vi "DestroyClone.vi"(8 "error in (no error)":errorcluster, 9 "Exit via Stop Module Req?":bool, 10 "Wait for Module to stop?":bool, 11 "ModuleAdmin":refnum<class "ModuleAdmin.lvclass">) -> (0 "error out":errorcluster, 1 "External Launch":bool, 3 "Mod Admin out":refnum<class "ModuleAdmin.lvclass">)   [LabVIEW 2014, in "PmuImpairModule.lvlib"]
uses:
  PmuImpairModule.lvlib
  <userlib>/NIST/ModuleAdminLib/ModuleAdmin/ModuleAdmin.lvclass
  <userlib>/NIST/ModuleAdminLib/ModuleAdmin/ModuleAdmin.lvclass/ModuleAdmin.ctl
  <userlib>/NIST/ModuleAdminLib/ModuleAdmin/Accessors/Read CloneRegRef.vi
  <userlib>/NIST/ModuleAdminLib/CloneRegistration/CloneRegistration.lvclass
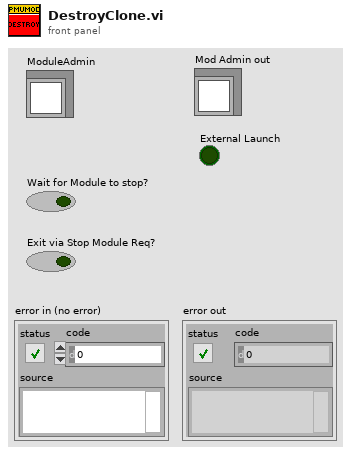
[diagram p1: front panel]
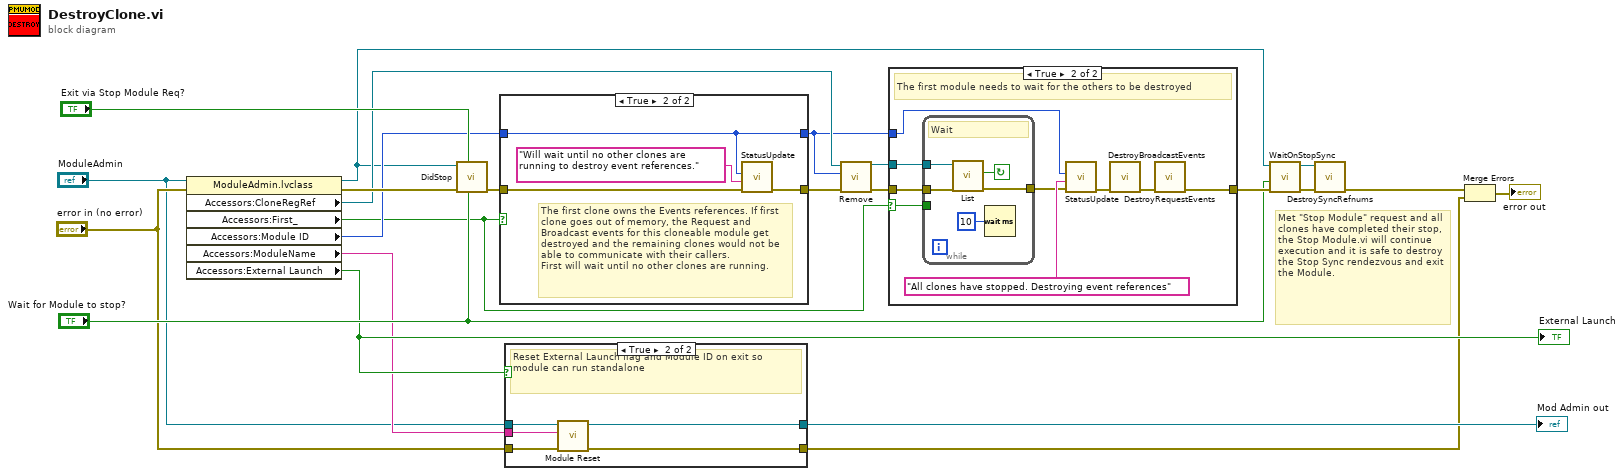
[diagram p0: block diagram]
diagram:
  # "Met \"Stop Module\" request and all clones have completed their stop, the Stop Module.vi will continue execution and it is safe to destroy the Stop Sync rendezvous and exit the Module."
  n1 = property class="ModuleAdmin.lvclass"(reference="ModuleAdmin", error in="error in (no error)") -> (reference out=w2:refnum<class "ModuleAdmin.lvclass">, error out=w23:errorcluster, "Accessors:CloneRegRef"=w3:refnum<data-value>, "Accessors:First_"=w4:bool, "Accessors:Module ID"=w7:i32, "Accessors:ModuleName"=w12:string, "Accessors:External Launch"=w14:bool)
  "External Launch" <- w14
  n2 = call "DidStop.vi"("Wait for Module to stop?"="Wait for Module to stop?", "Exit via Stop Module Req?"="Exit via Stop Module Req?", "error in (no error)"=w23, "ModuleAdmin"=w2) -> ("error out"=w21:errorcluster)  [unwired: 7 in]
  n3 = case shown="True" w4 {
    tunnel: w21 -> [w25 w29]
    tunnel: w7 -> [w24 w26]
    tunnel: [w25 w27] -> w20
    tunnel: [w24 w26] -> w1
    frame False {
    }
    frame True {
      # "The first clone owns the Events references. If first clone goes out of memory, the Request and Broadcast events for this cloneable module get destroyed and the remaining clones would not be able to communicate with their callers.\nFirst will wait until no other clones are running."
      n4 = call "StatusUpdate.vi"("error in (no error)"=w29, "Status"="Will wait until no other clones are running to destroy event references." ("format string"), "ModuleID"=w26) -> ("error out"=w27:errorcluster)  [unwired: 8 in]
    }
  }
  n5 = case shown="True" w14 {
    tunnel: "error in (no error)" -> [w30 w36]
    tunnel: w12 -> [_ w35]
    tunnel: "ModuleAdmin" -> [w31 w34]
    tunnel: [w31 w33] -> w10
    tunnel: [w30 w32] -> w8
    frame False {
    }
    frame True {
      # "Reset External Launch flag and Module ID on exit so module can run standalone"
      n6 = call <userlib>:"Module Reset.vi"("error in (no error)"=w36, "ModuleName"=w35, "Mod Admin in"=w34) -> ("error out"=w32:errorcluster, "Mod Admin out"=w33:refnum<class "ModuleAdmin.lvclass">)  [unwired: 7 in]
    }
  }
  "Mod Admin out" <- w10
  n7 = call <userlib>:"Remove.vi"("error in (no error)"=w20, "Module ID"=w1, "CloneRegRef"=w3) -> ("error out"=w19:errorcluster, "CloneRegRef"=w6:refnum<data-value>)  [unwired: 6 in, 1 out]
  n8 = case shown="True" w4 {
    selector: w4 -> [_ w45]
    tunnel: w19 -> [w37 w46]
    tunnel: w1 -> [_ w39]
    tunnel: [w37 w40] -> w18
    tunnel: w6 -> [_ w38]
    frame False {
    }
    frame True {
      # "The first module needs to wait for the others to be destroyed"
      n9 = while {
        tunnel: w46 -> [w51]
        tunnel: w45 -> [_]
        tunnel: [w50] -> w43
        tunnel: w38 -> [w47]
        stop <- w48 continue-if-true
        # "Wait"
        n10 = call <userlib>:"List.vi"("error in (no error)"=w51, "CloneRegRef"=w47) -> ("error out"=w50:errorcluster, "Found?"=w48:bool)  [unwired: 4 in, 4 out]
        n11 = Wait (ms)(milliseconds to wait=u32 10) -> ()  [unwired: 1 out]
      }
      n12 = call "StatusUpdate.vi"("error in (no error)"=w43, "Status"="All clones have stopped. Destroying event references", "ModuleID"=w39) -> ("error out"=w42:errorcluster)  [unwired: 8 in]
      n13 = call "DestroyBroadcastEvents.vi"("error in (no error)"=w42) -> ("error out"=w41:errorcluster)  [unwired: 10 in]
      n14 = call "DestroyRequestEvents.vi"("error in (no error)"=w41) -> ("error out"=w40:errorcluster)  [unwired: 10 in]
    }
  }
  n15 = call <userlib>:"WaitOnStopSync.vi"("error in (no error)"=w18, "WaitForModuleToStop?"="Wait for Module to stop?", "ModuleAdmin"=w2) -> ("error out"=w16:errorcluster, "ModuleAdmin"=w5:refnum<class "ModuleAdmin.lvclass">)  [unwired: 7 in]
  n16 = call <userlib>:"DestroySyncRefnums.vi"("error in (no error)"=w16, "ModuleAdmin"=w5) -> ("error out"=w15:errorcluster)  [unwired: 9 in]
  n17 = Merge Errors(w15, w8) -> (→"error out":errorcluster)
